vi "多参数状态告警table定义.vi"(7 "table输入":string, 11 "data":T2) -> (1 "table输出":string, 2 "columns":string[](array[string]), 3 "data 输出":T1)   [LabVIEW 2016, in "database.lvlib"]
uses:
  database.lvlib
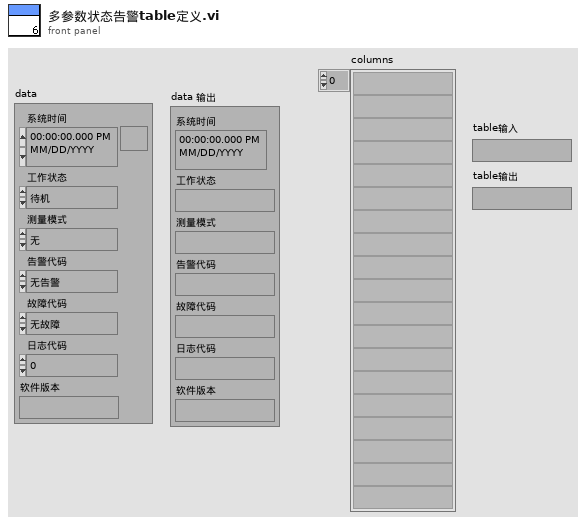
[diagram p1: front panel]
types:
  T1 = cluster{"系统时间":timestamp, "工作状态":string, "测量模式":string, "告警代码":string, "故障代码":string, "日志代码":string, "软件版本":string}
  T2 = cluster{"系统时间":timestamp, "工作状态":enum16{"待机", "启动测量", "标样核查", "零点核查", "跨度核查", "空白测试", "平行样测试", "加标回收", "空白校准", "标样校准", "初始化（清洗）", "停止测试", "仪器重启", "校时", "模式设置", "测量间隔设置", "零点核查间隔设置", "跨度核查间隔设置", "标样核查间隔设置"}, "测量模式":enum16{"无", "连续模式", "周期模式", "定点模式", "受控模式", "手动模式"}, "告警代码":enum16{"无告警", "缺试剂告警", "缺水样告警", "缺蒸馏水告警", "缺标液告警", "仪表漏液告警", "标定异常告警", "超量程告警", "加热异常", "低试剂预警", "超上限告警", "超下限告警", "仪表内部其他异常", "滴定异常告警", "电极异常告警", "量程切换告警", "参数设置告警", "PH电极电位异常", "电导率电极异常", "浊度光度异常", "溶解氧电极异常", "溶解氧光强异常", "温度异常告警", "PH异常告警", "溶解氧异常告警", "电导率异常告警", "浊度异常告警", "叶绿素异常告警", "藻密度异常告警", "蓝绿藻异常告警", "ORP异常告警", "氨氮异常告警", "清洁刷异常告警", "SD卡异常告警", "蓝牙异常告警", "Wifi异常告警", "流程异常告警"}, "故障代码":enum16{"无故障", "电机故障", "温度故障", "通讯故障", "滴定故障"}, "日志代码":u16, "软件版本":string}
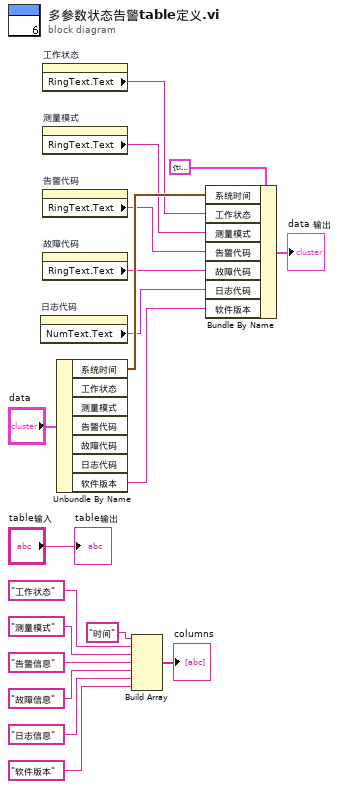
[diagram p0: block diagram]
diagram:
  n1 = property on="日志代码" class="DigNum (严格)"() -> ("NumText.Text"=w3:string)  [unwired: 2 in, 2 out]
  n2 = property on="工作状态" class="Enum (严格)"() -> ("RingText.Text"=w7:string)  [unwired: 2 in, 2 out]
  n3 = property on="测量模式" class="Enum (严格)"() -> ("RingText.Text"=w6:string)  [unwired: 2 in, 2 out]
  n4 = property on="告警代码" class="Enum (严格)"() -> ("RingText.Text"=w5:string)  [unwired: 2 in, 2 out]
  n5 = property on="故障代码" class="Enum (严格)"() -> ("RingText.Text"=w4:string)  [unwired: 2 in, 2 out]
  n6 = Unbundle By Name("data") -> ("系统时间"=w9:timestamp, "软件版本"=w1:string)  [unwired: 5 out]
  n7 = Build Array("时间", "工作状态", "测量模式", "告警信息", "故障信息", "日志信息", "软件版本") -> (→"columns":string[])
  n8 = Bundle By Name(cluster=T1 {"系统时间"=timestamp(0 s since 1904-01-01), "工作状态"="", "测量模式"="", "告警代码"="", "故障代码"="", "日志代码"="", "软件版本"=""} ("data 输出"), "系统时间"=w9, "工作状态"=w7, "测量模式"=w6, "告警代码"=w5, "故障代码"=w4, "日志代码"=w3, "软件版本"=w1) -> (→"data 输出":T1)
  "table输出" <- "table输入"
